vi "config.vi"() -> (3 "save ok":bool)   [LabVIEW 2016]
uses:
  <vilib>/Analysis/baseanly.llb/Mean (DBL).vi
  <vilib>/gmath/NI_Gmath.lvlib
  <vilib>/Analysis/NI_AALBase.lvlib
panel:
  out "Strain ini":cluster{"Strain ini":dbl[]}
  in  "Save":cluster{"Save Path":path, "File Name":string}
  in  "Resistor Set":T1={"Criterion Level"=1000.0, "Res. Set"=[{"Res. Ch"=1.0, "Res. Active"=TRUE, "Res Initial"=0.0}]}
  in  "Close":bool
  in  "Save":bool
  in  "Open":bool
  in  "Test Stop Condition":T2={"Test cycle"=1, "Fail number in a cycle"=0, "Fail factor"={"Duration"=0, "Fail No."=0}} {"Fail factor"."Fail No." min=1 max=60000; "Fail factor"."Duration" min=1 max=60000; "Test cycle" min=1 max=60000}
  in  "Acceleration Condition":T3={"Shock duration pecent [%]"=10, "Filter cutoff freq"=5000} {"Shock duration pecent [%]" min=1 max=99 format="%#.0f"}
  in  "Get Res.":bool
  in  "Sensor Test":bool
  in  "Sensor Set":T4={"Accelerometer"={"Sensitivity(mV/g)"=10.0}, "Strain Guage"={"Ch."=[1.0, 2.0, 3.0, 4.0], "Gage factor"=[2.0, 2.0, 2.0, 2.0], "Resistance"=[120.0, 120.0, 120.0, 120.0], "Poisson ratio"=[]}}
  in  "Get Time":bool
  in  "Test Info":T5={"date"="16-01-20, 10:52:59", "custom"="", "oper"="", "package"="", "pkg side"="", "solder"="", "brd side"="", "paste"="", "reflow"=""}
  out "Deco":bool
  # "Configuration"
  # "Select    Ch.    Initial"
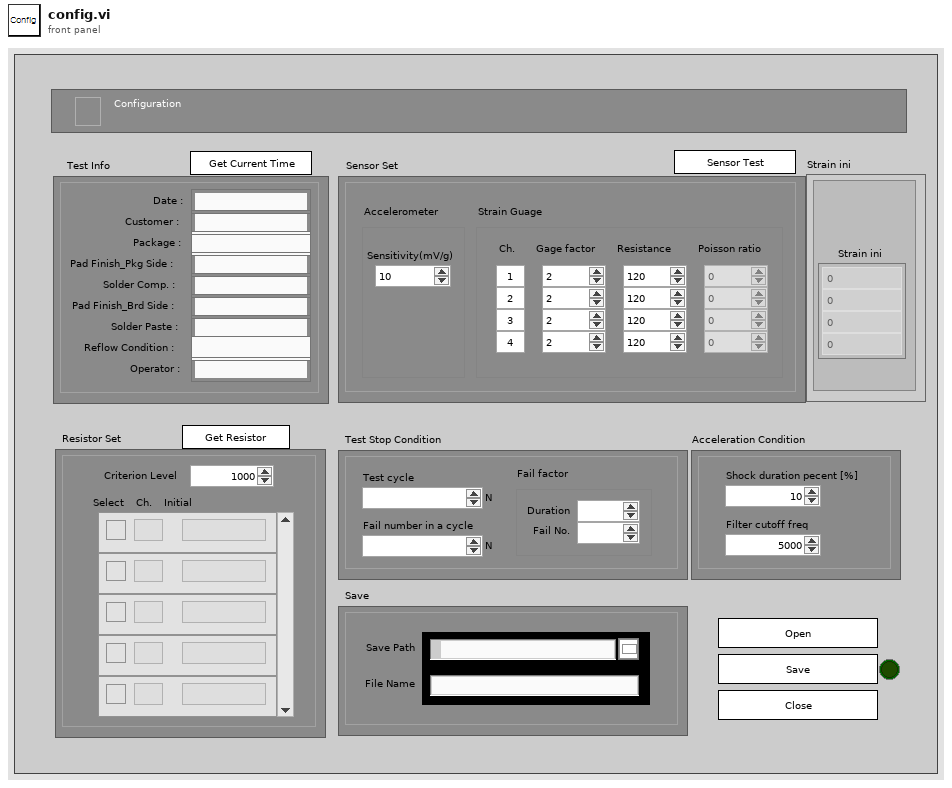
[diagram p1: front panel]
types:
  T1 = cluster{"Criterion Level":dbl, "Res. Set":cluster{"Res. Ch":dbl, "Res. Active":bool, "Res Initial":dbl}[]}
  T2 = cluster{"Test cycle":u16, "Fail number in a cycle":u16, "Fail factor":cluster{"Duration":u16, "Fail No.":u16}}
  T3 = cluster{"Shock duration pecent [%]":u16, "Filter cutoff freq":u32}
  T4 = cluster{"Accelerometer":cluster{"Sensitivity(mV/g)":dbl}, "Strain Guage":cluster{"Ch.":dbl[], "Gage factor":dbl[], "Resistance":dbl[], "Poisson ratio":dbl[]}}
  T5 = cluster{"date":string, "custom":string, "oper":string, "package":string, "pkg side":string, "solder":string, "brd side":string, "paste":string, "reflow":string}
  T6 = cluster{"Test Information":cluster{"date":string, "custom":string, "oper":string, "package":string, "pkg side":string, "solder":string, "brd side":string, "paste":string, "reflow":string}, "Sensor Set":cluster{"Accelerometer":cluster{"Sensitivity(mV/g)":dbl}, "Strain Guage":cluster{"Ch.":dbl[], "Gage factor":dbl[], "Resistance":dbl[], "Poisson ratio":dbl[]}}, "Resistor Set":cluster{"Criterion Level":dbl, "Res. Set":cluster{"Res. Ch":dbl, "Res. Active":bool, "Res Initial":dbl}[]}, "Test Stop Condition":cluster{"Test cycle":u16, "Fail number in a cycle":u16, "Fail factor":cluster{"Duration":u16, "Fail No.":u16}}, "Acceleration Condition ":cluster{"Shock duration pecent [%]":u16, "Filter cutoff freq":u32}, "Save":cluster{"Save Path":path, "File Name":string}}
  T7 = cluster{"Res. Ch":dbl, "Res. Active":bool, "Res Initial":dbl}
  T8 = enum16{"Config Save", "Config Load", "LastRUN Save", "LastRUN Load"}
  T9 = enum16{"arithmetic", "geometric", "harmonic", "trimmed", "median"}
  T10 = cluster{"Res. Ch":dbl, "Res. Active":bool, "Res Initial":dbl}[]
  T11 = cluster{"Test Information":cluster{"date":string, "custom":string, "oper":string, "package":string, "pkg side":string, "solder":string, "brd side":string, "paste":string, "reflow":string}, "Sensor Set":cluster{"Accelerometer":cluster{"Sensitivity(mV/g)":dbl}, "Strain Guage":cluster{"Ch.":dbl[], "Gage factor":dbl[], "Resistance":dbl[], "Poisson ratio":dbl[]}}, "Resistor Set":cluster{"Criterion Level":dbl, "Res. Set":cluster{"Res. Ch":dbl, "Res. Active":bool, "Res Initial":dbl}[]}, "Test Stop Condition":cluster{"Test cycle":u16, "Fail number in a cycle":u16, "Fail factor":cluster{"Duration":u16, "Fail No.":u16}}, "Acceleration Condition":cluster{"Shock duration pecent [%]":u16, "Filter cutoff freq":u32}, "Save":cluster{"Save Path":path, "File Name":string}}
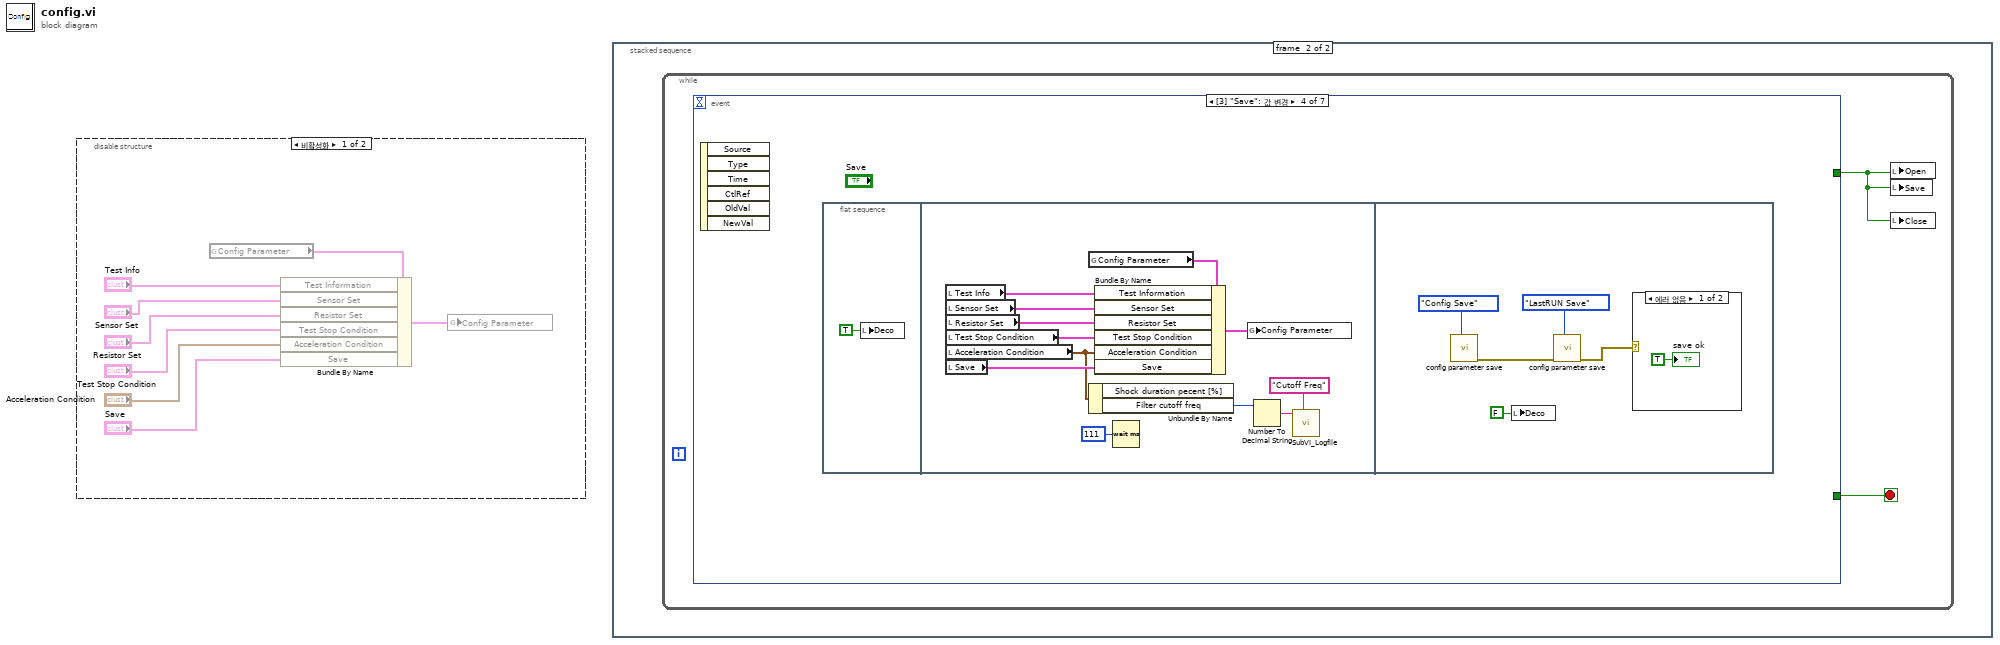
[diagram p0: block diagram]
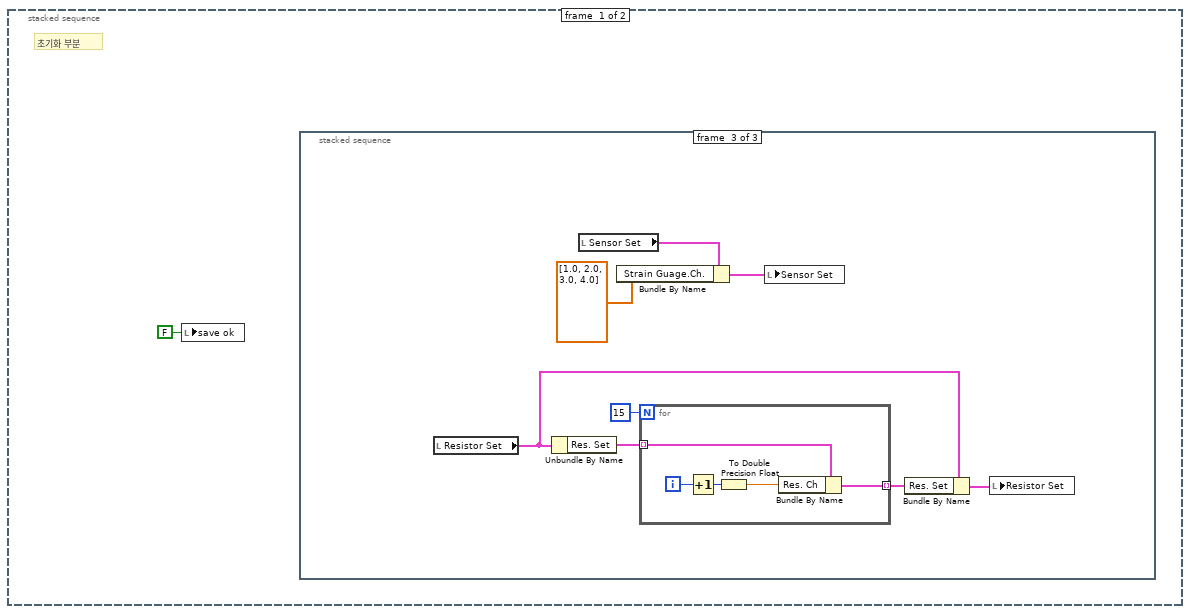
[diagram p2: hidden frame]
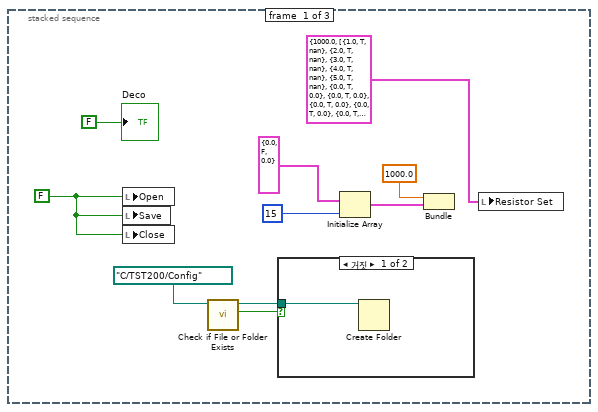
[diagram p3: hidden frame]
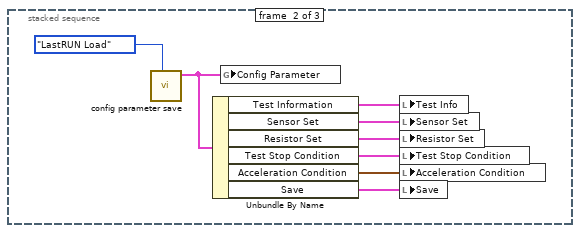
[diagram p5: hidden frame]
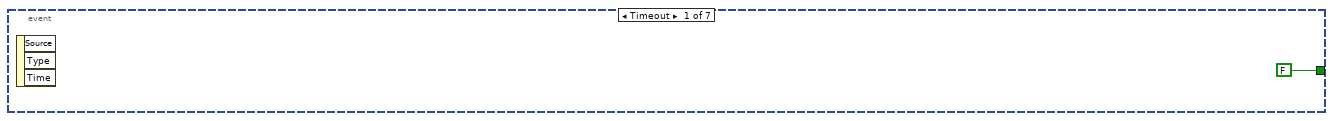
[diagram p6: hidden frame]
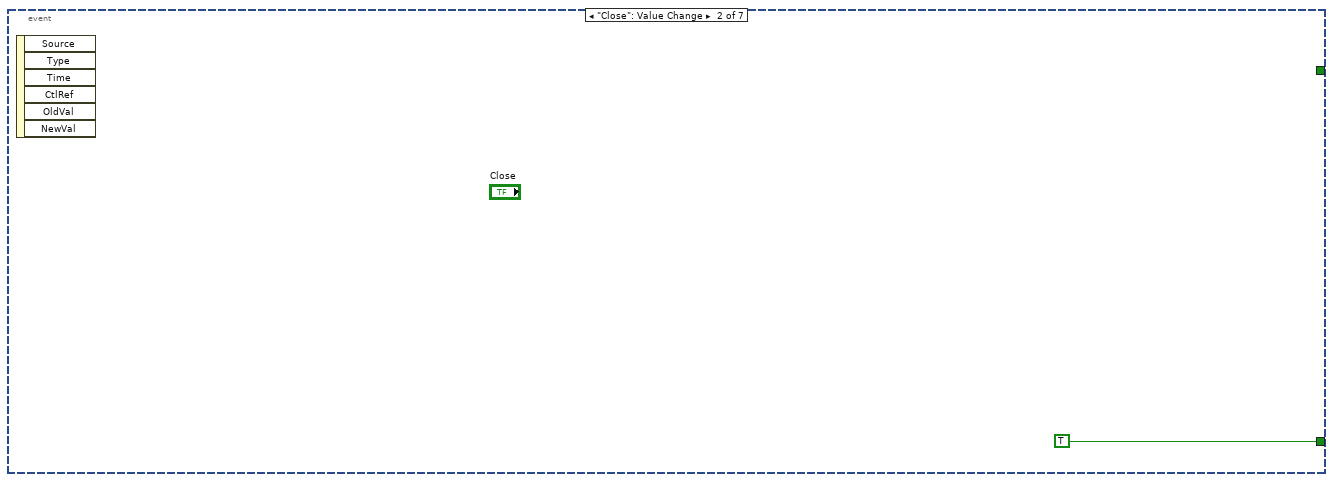
[diagram p7: hidden frame]
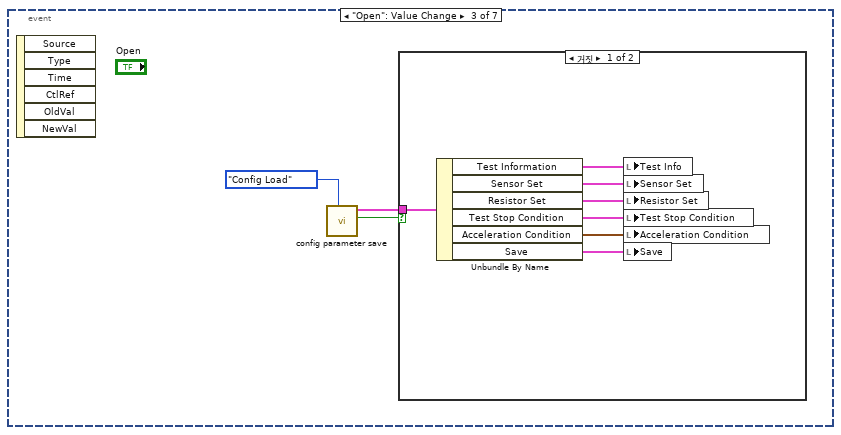
[diagram p8: hidden frame]
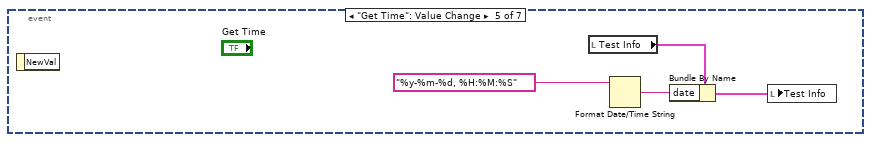
[diagram p11: hidden frame]
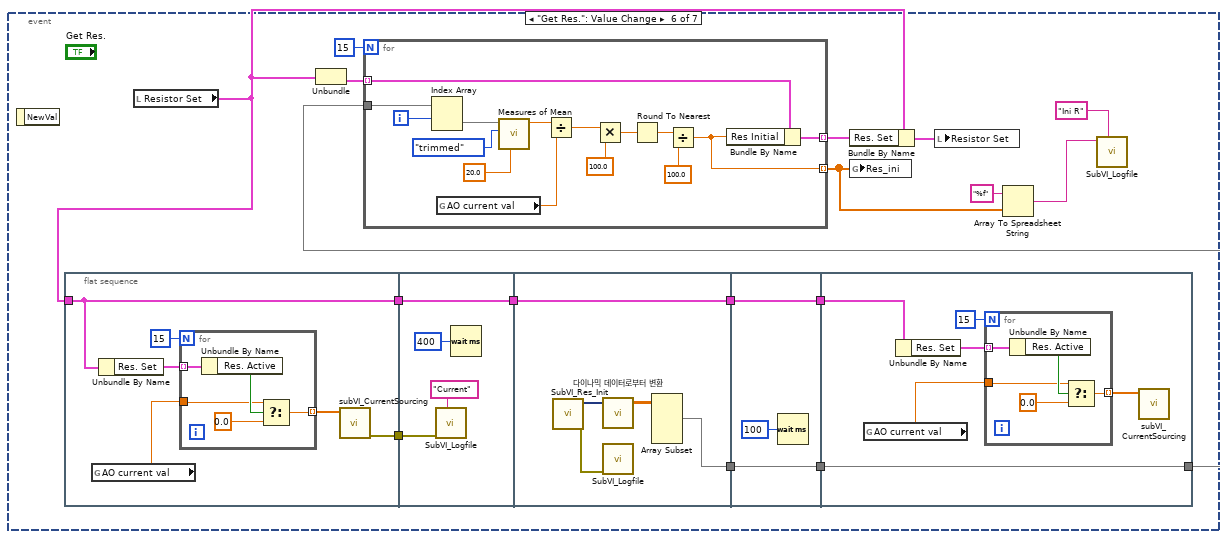
[diagram p12: hidden frame]
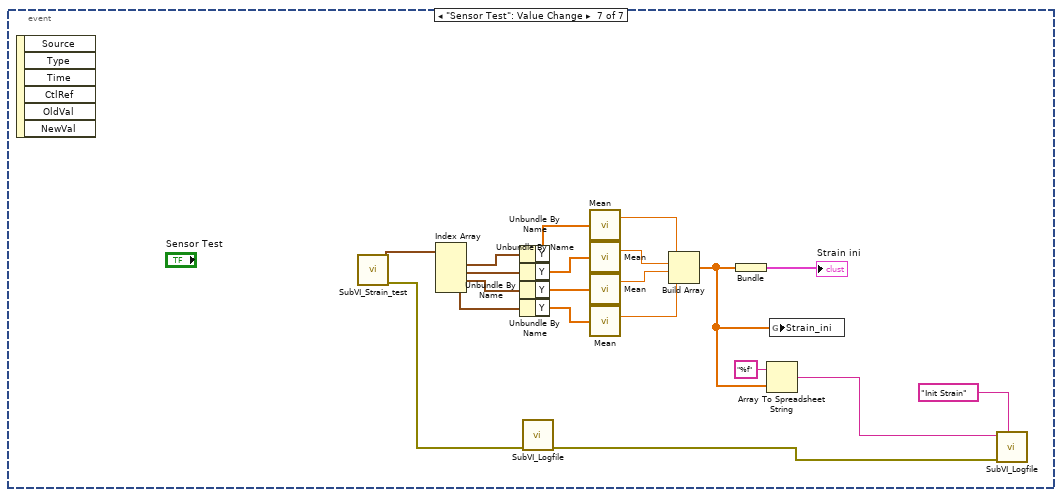
[diagram p13: hidden frame]
diagram:
  n1 = disable-structure shown="비활성화" {
    frame Disabled {
      n2 = global read "글로벌_Config Parameter.vi" "Config Parameter"() -> (w8:T6)
      n3 = Bundle By Name(cluster=w8, "Test Information"="Test Info", "Sensor Set"="Sensor Set", "Resistor Set"="Resistor Set", "Test Stop Condition"="Test Stop Condition", "Acceleration Condition"="Acceleration Condition", "Save"="Save") -> (w1:T6)
      n4 = global write "글로벌_Config Parameter.vi" "Config Parameter"(w1) -> ()
    }
    frame Enabled {
    }
  }
  n5 = stacked-sequence {
    frame #0 {
      # "초기화 부분"
      n6 = local write "save ok"(FALSE ("save ok")) -> ()
      n7 = stacked-sequence {
        frame #0 {
          w15 = FALSE ("Open")
          n8 = local write "Open"(w15) -> ()
          n9 = local write "Save"(w15) -> ()
          n10 = local write "Close"(w15) -> ()
          n11 = call <vilib>:"Check if File or Folder Exists.vi"("path"=path "C:/TST200/Config" ("XML File Path")) -> ("file or folder exists?"=w12:bool, "dup path"=w11:path)  [unwired: 8 in, 1 out]
          n12 = case shown="거짓" w12 {
            tunnel: w11 -> [w20 _]
            frame False {
              n13 = Create Folder(path (use dialog)=w20) -> ()  [unwired: 2 in, 3 out]
            }
            frame True {
            }
          }
          n14 = Initialize Array(T7 {"Res. Ch"=0.0, "Res. Active"=FALSE, "Res Initial"=0.0} ("Res Set"), 15 ("차원 크기")) -> (w19:T10)
          n15 = Bundle("Criterion Level"=1000.0, w19) -> ()  [unwired: 1 in, 1 out]
          n16 = local write "Resistor Set"(T1 {"Criterion Level"=1000.0, "Res. Set"=[{"Res. Ch"=1.0, "Res. Active"=TRUE, "Res Initial"=nan}, {"Res. Ch"=2.0, "Res. Active"=TRUE, "Res Initial"=nan}, {"Res. Ch"=3.0, "Res. Active"=TRUE, "Res Initial"=nan}, {"Res. Ch"=4.0, "Res. Active"=TRUE, "Res Initial"=nan}, {"Res. Ch"=5.0, "Res. Active"=TRUE, "Res Initial"=nan}, {"Res. Ch"=0.0, "Res. Active"=TRUE, "Res Initial"=0.0}, {"Res. Ch"=0.0, "Res. Active"=TRUE, "Res Initial"=0.0}, {"Res. Ch"=0.0, "Res. Active"=TRUE, "Res Initial"=0.0}, {"Res. Ch"=0.0, "Res. Active"=TRUE, "Res Initial"=0.0}, {"Res. Ch"=0.0, "Res. Active"=TRUE, "Res Initial"=0.0}, {"Res. Ch"=0.0, "Res. Active"=TRUE, "Res Initial"=0.0}, {"Res. Ch"=0.0, "Res. Active"=TRUE, "Res Initial"=0.0}, {"Res. Ch"=0.0, "Res. Active"=TRUE, "Res Initial"=0.0}, {"Res. Ch"=0.0, "Res. Active"=TRUE, "Res Initial"=0.0}, {"Res. Ch"=0.0, "Res. Active"=TRUE, "Res Initial"=0.0}]} ("Resistor Set 2")) -> ()
          "Deco" <- FALSE ("deco")
        }
        frame #1 {
          n17 = call "config parameter save.vi"("ctl"=T8."LastRUN Load") -> ("Config Parameter 2"=w22:T11)  [unwired: 8 in, 2 out]
          n18 = Unbundle By Name(w22) -> ("Test Information"=w23:T5, "Sensor Set"=w24:T4, "Resistor Set"=w25:T1, "Test Stop Condition"=w26:T2, "Acceleration Condition"=w27:T3, "Save"=w28:cluster{"Save Path":path, "File Name":string})
          n19 = global write "글로벌_Config Parameter.vi" "Config Parameter"(w22) -> ()
          n20 = local write "Test Info"(w23) -> ()
          n21 = local write "Sensor Set"(w24) -> ()
          n22 = local write "Resistor Set"(w25) -> ()
          n23 = local write "Test Stop Condition"(w26) -> ()
          n24 = local write "Acceleration Condition"(w27) -> ()
          n25 = local write "Save"(w28) -> ()
        }
        frame #2 {
          n26 = local read "Resistor Set"() -> (w33:T1)
          n27 = Unbundle By Name(w33) -> ("Res. Set"=w31:T10)
          n28 = local read "Sensor Set"() -> (w36:T4)
          n29 = Bundle By Name(cluster=w36, "Strain Guage.Ch."=dbl[] [1.0, 2.0, 3.0, 4.0]) -> (w30:T4)
          n30 = for {
            N: 15 -> [_]
            tunnel: w31 -> [w41] mode=indexing
            tunnel: [w37] -> w34 mode=indexing
            i -> [w40]
            n31 = Increment(x=w40) -> (x+1=w39:i32)
            n32 = To Double Precision Float(number=w39) -> (double precision float=w38:dbl)
            n33 = Bundle By Name(cluster=w41, "Res. Ch"=w38) -> (w37:T7)
          }
          n34 = local write "Sensor Set"(w30) -> ()
          n35 = Bundle By Name(cluster=w33, "Res. Set"=w34) -> (w29:T1)
          n36 = local write "Resistor Set"(w29) -> ()
        }
      }
    }
    frame #1 {
      n37 = while {
        stop <- w42 stop-if-true
        n38 = event shown="[3] \"Save\": 값 변경" {
          selector: _ -> [_ _ _ _ _ _ _]
          dyn-events: _ -> [_ _ _ _ _ _ _]
          timeout: _ -> [_ _ _ _ _ _ _]
          tunnel: [FALSE ("Open") _ _ _ _ _ _] -> w43
          tunnel: [_ TRUE _ _ _ _ _] -> w42
          event Timeout {
            n39 = event-data() -> ()  [unwired: 1 in, 3 out]
          }
          event "Close": Value Change {
            n40 = event-data() -> ()  [unwired: 1 in, 6 out]
          }
          event "Open": Value Change {
            n41 = event-data() -> ()  [unwired: 1 in, 6 out]
            n42 = call "config parameter save.vi"("ctl"=T8."Config Load") -> ("open cancelled"=w47:bool, "Config Parameter 2"=w46:T11)  [unwired: 8 in, 1 out]
            n43 = case shown="거짓" w47 {
              tunnel: w46 -> [w49 _]
              frame False {
                n44 = Unbundle By Name(w49) -> ("Test Information"=w50:T5, "Sensor Set"=w51:T4, "Resistor Set"=w52:T1, "Test Stop Condition"=w53:T2, "Acceleration Condition"=w54:T3, "Save"=w55:cluster{"Save Path":path, "File Name":string})
                n45 = local write "Test Info"(w50) -> ()
                n46 = local write "Sensor Set"(w51) -> ()
                n47 = local write "Resistor Set"(w52) -> ()
                n48 = local write "Test Stop Condition"(w53) -> ()
                n49 = local write "Acceleration Condition"(w54) -> ()
                n50 = local write "Save"(w55) -> ()
              }
              frame True {
              }
            }
          }
          event "Save": Value Change {
            n51 = event-data() -> ()  [unwired: 1 in, 6 out]
            n52 = flat-sequence {
              frame #0 {
                n53 = local write "Deco"(TRUE ("Deco")) -> ()
              }
              frame #1 {
                n54 = local read "Test Info"() -> (w67:T5)
                n55 = local read "Sensor Set"() -> (w66:T4)
                n56 = local read "Resistor Set"() -> (w65:T1)
                n57 = local read "Test Stop Condition"() -> (w64:T2)
                n58 = local read "Acceleration Condition"() -> (w58:T3)
                n59 = local read "Save"() -> (w63:cluster{"Save Path":path, "File Name":string})
                n60 = global read "글로벌_Config Parameter.vi" "Config Parameter"() -> (w68:T6)
                n61 = Unbundle By Name(w58) -> ("Filter cutoff freq"=w57:u32)  [unwired: 1 out]
                n62 = Bundle By Name(cluster=w68, "Test Information"=w67, "Sensor Set"=w66, "Resistor Set"=w65, "Test Stop Condition"=w64, "Acceleration Condition"=w58, "Save"=w63) -> (w61:T6)
                n63 = Wait (ms)(milliseconds to wait=u32 111 ("대기 시간(ms)")) -> ()  [unwired: 1 out]
                n64 = global write "글로벌_Config Parameter.vi" "Config Parameter"(w61) -> ()
                n65 = Number To Decimal String(number=w57) -> (decimal integer string=w60:string)  [unwired: 1 in]
                n66 = call "SubVI_Logfile.vi"("Title"="Cutoff Freq", "desc"=w60) -> ()  [unwired: 9 in, 1 out]
              }
              frame #2 {
                n67 = call "config parameter save.vi"("ctl"=T8."Config Save") -> ("error out"=w72:errorcluster)  [unwired: 8 in, 2 out]
                n68 = local write "Deco"(FALSE ("Deco")) -> ()
                n69 = call "config parameter save.vi"("ctl"=T8."LastRUN Save", "error in"=w72) -> ("error out"=w69:errorcluster)  [unwired: 7 in, 2 out]
                n70 = case shown="에러 없음" w69 {
                  frame No Error {
                    "save ok" <- TRUE ("save ok")
                  }
                  frame Error {
                  }
                }
              }
            }
          }
          event "Get Time": Value Change {
            n71 = event-data() -> ()  [unwired: 1 in, 1 out]
            n72 = local read "Test Info"() -> (w77:T5)
            n73 = Format Date/Time String(time format string (%c)="%y-%m-%d, %H:%M:%S") -> (date/time string=w76:string)  [unwired: 2 in]
            n74 = Bundle By Name(cluster=w77, "date"=w76) -> (w75:T5)
            n75 = local write "Test Info"(w75) -> ()
          }
          event "Get Res.": Value Change {
            n76 = event-data() -> ()  [unwired: 1 in, 1 out]
            n77 = flat-sequence {
              tunnel: w92 -> [w100]
              tunnel: [w100] -> w85
              tunnel: [w96] -> w83
              tunnel: [w109] -> w86
              tunnel: w85 -> [w109]
              tunnel: w83 -> [w108]
              tunnel: [w113] -> w89
              tunnel: [w112] -> w87
              tunnel: w86 -> [w112]
              tunnel: [w117] -> w90
              tunnel: w89 -> [w117]
              tunnel: [w116] -> w88
              tunnel: w87 -> [w116]
              tunnel: [w123] -> w91
              tunnel: w90 -> [w123]
              tunnel: w88 -> [w122]
              frame #0 {
                n78 = global read "글로벌_Config Parameter.vi" "AO current val"() -> (w97:dbl)
                n79 = Unbundle By Name(w100) -> ("Res. Set"=w101:T10)
                n80 = for {
                  N: 15 -> [_]
                  tunnel: [w102] -> w99 mode=indexing
                  tunnel: w97 -> [w104]
                  tunnel: w101 -> [w106] mode=indexing
                  n81 = Unbundle By Name(w106) -> ("Res. Active"=w105:bool)
                  n82 = Select(t=w104, s=w105, f=0.0 ("데이터")) -> (s? t:f=w102:dbl)
                }
                n83 = call "subVI_CurrentSourcing.vi"("Curr set val"=w99) -> ("error out"=w96:errorcluster)  [unwired: 5 in, 1 out]
              }
              frame #1 {
                n84 = call "SubVI_Logfile.vi"("Title"="Current", "error in"=w108) -> ()  [unwired: 9 in, 1 out]
                n85 = Wait (ms)(milliseconds to wait=u32 400 ("대기 시간(ms)")) -> ()  [unwired: 1 out]
              }
              frame #2 {
                n86 = call "SubVI_Res_Init.vi"() -> ("error out"=w111:errorcluster, "data"=w114:dynamicdata)  [unwired: 10 in]
                n87 = call "다이나믹 데이터로부터 변환"("Dynamic Data Type"=w114) -> ("Array"=w115:dbl[][])  [unwired: 3 in]
                n88 = call "SubVI_Logfile.vi"("error in"=w111) -> ()  [unwired: 10 in, 1 out]
                n89 = Array Subset(array=w115) -> (w113:dbl[][])  [unwired: 4 in]
              }
              frame #3 {
                n90 = Wait (ms)(milliseconds to wait=u32 100 ("대기 시간(ms)")) -> ()  [unwired: 1 out]
              }
              frame #4 {
                n91 = global read "글로벌_Config Parameter.vi" "AO current val"() -> (w119:dbl)
                n92 = Unbundle By Name(w122) -> ("Res. Set"=w124:T10)
                n93 = for {
                  N: 15 -> [_]
                  tunnel: [w125] -> w121 mode=indexing
                  tunnel: w119 -> [w127]
                  tunnel: w124 -> [w129] mode=indexing
                  n94 = Unbundle By Name(w129) -> ("Res. Active"=w128:bool)
                  n95 = Select(t=w127, s=w128, f=0.0 ("데이터")) -> (s? t:f=w125:dbl)
                }
                n96 = call "subVI_CurrentSourcing.vi"("Curr set val"=w121) -> ()  [unwired: 5 in, 2 out]
              }
            }
            n97 = local read "Resistor Set"() -> (w92:T1)
            n98 = Unbundle(w92) -> ("Res. Set"=w95:T10)  [unwired: 1 out]
            n99 = for {
              N: 15 -> [_]
              tunnel: w91 -> [w144]
              tunnel: w95 -> [w139] mode=indexing
              tunnel: [w138] -> w94 mode=indexing
              tunnel: [w131] -> w82 mode=indexing
              i -> [w143]
              n100 = Index Array(array=w144, index (row)=w143) -> (element=w142:dbl[])  [unwired: 1 in]
              n101 = global read "글로벌_Config Parameter.vi" "AO current val"() -> (w130:dbl)
              n102 = call <vilib>:"Measures of Mean.vi"("percent (trim)"=20.0, "type"=T9."trimmed", "x array"=w142) -> ("mean value"=w137:dbl)  [unwired: 7 in, 1 out]
              n103 = Divide(x=w137, y=w130) -> (x/y=w136:dbl)
              n104 = Multiply(x=w136, y=100.0) -> (x*y=w134:dbl)
              n105 = Round To Nearest(number=w134) -> (nearest integer value=w133:dbl)
              n106 = Divide(x=w133, y=100.0) -> (x/y=w131:dbl)
              n107 = Bundle By Name(cluster=w139, "Res Initial"=w131) -> (w138:T7)
            }
            n108 = Bundle By Name(cluster=w92, "Res. Set"=w94) -> (w93:T1)
            n109 = global write "글로벌_Config Parameter.vi" "Res_ini"(w82) -> ()
            n110 = local write "Resistor Set"(w93) -> ()
            n111 = Array To Spreadsheet String(array=w82, 3:"%f" ("포맷 문자열")) -> (spreadsheet string=w80:string)  [unwired: 1 in]
            n112 = call "SubVI_Logfile.vi"("Title"="Ini R", "desc"=w80) -> ()  [unwired: 9 in, 1 out]
          }
          event "Sensor Test": Value Change {
            n113 = event-data() -> ()  [unwired: 1 in, 6 out]
            n114 = call "SubVI_Strain_test.vi"() -> ("error out"=w150:errorcluster, "웨이브폼 차트"=w164:waveform(dbl)[])  [unwired: 10 in]
            n115 = Index Array(array=w164) -> (element #1=w163:waveform(dbl), element #2=w160:waveform(dbl), element #3=w161:waveform(dbl), element #4=w162:waveform(dbl))  [unwired: 4 in]
            n116 = Unbundle By Name(w163) -> ("Y"=w159:dbl[])
            n117 = Unbundle By Name(w160) -> ("Y"=w158:dbl[])
            n118 = Unbundle By Name(w161) -> ("Y"=w157:dbl[])
            n119 = Unbundle By Name(w162) -> ("Y"=w156:dbl[])
            n120 = call "SubVI_Logfile.vi"("error in"=w150) -> ("error out"=w149:errorcluster)  [unwired: 10 in]
            n121 = call-poly <vilib>:"Mean.vi"("X"=w159) -> ("mean"=w155:dbl)  [unwired: 1 out]
            n122 = call-poly <vilib>:"Mean.vi"("X"=w158) -> ("mean"=w153:dbl)  [unwired: 1 out]
            n123 = call-poly <vilib>:"Mean.vi"("X"=w157) -> ("mean"=w152:dbl)  [unwired: 1 out]
            n124 = call-poly <vilib>:"Mean.vi"("X"=w156) -> ("mean"=w154:dbl)  [unwired: 1 out]
            n125 = Build Array(w155, w153, w152, w154) -> (w146:dbl[])
            n126 = Bundle(w146) -> (→"Strain ini":cluster{dbl[]})  [unwired: 1 in]
            n127 = Array To Spreadsheet String(array=w146, 3:"%f" ("포맷 문자열")) -> (spreadsheet string=w147:string)  [unwired: 1 in]
            n128 = global write "글로벌_Config Parameter.vi" "Strain_ini"(w146) -> ()
            n129 = call "SubVI_Logfile.vi"("Title"="Init Strain", "error in"=w149, "desc"=w147) -> ()  [unwired: 8 in, 1 out]
          }
        }
        n130 = local write "Open"(w43) -> ()
        n131 = local write "Save"(w43) -> ()
        n132 = local write "Close"(w43) -> ()
      }
    }
  }
